vi "getYGAP.vi"(0 "reference":refnum<class "CallNode.lvclass">, 5 "error in (no error)":errorcluster) -> (14 "reference out":refnum<class "CallNode.lvclass">, 15 "CALL_YGAP":i32, 19 "error out":errorcluster)   [LabVIEW 2020, in "CallNode.lvclass"]
doc: "Gets the public YGAP values"
uses:
  <resource>/Framework/Providers/Open_GDS/UML/CallNode_class/CallNode.lvclass
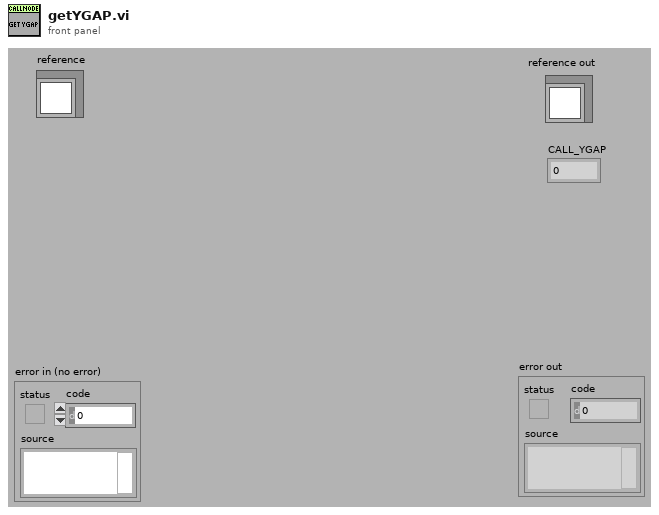
[diagram p1: front panel]
types:
  T1 = typedef "CallNode.lvclass/ClassAttributes.ctl" = cluster{"Base class":T2, "CALL_YGAP":i32}
  T2 = typedef "RectangularNode.lvclass/ClassAttributes.ctl" = cluster{"Base class":T3, "childClassAttribute2":enum16{"Hello", "Goodbye"}}
  T3 = typedef "AbstractNode.lvclass/ClassAttributes.ctl" = cluster{"classAttribute1":bool}
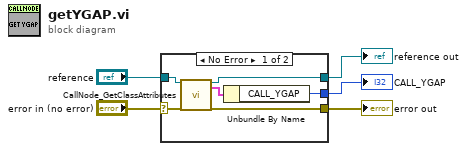
[diagram p0: block diagram]
diagram:
  n1 = case shown="No Error" "error in (no error)" {
    selector: "error in (no error)" -> [w11 w12]
    tunnel: "reference" -> [w10 w13]
    tunnel: [w8 w12] -> w3
    tunnel: [w9 w13] -> w2
    tunnel: [w7 _] -> w1
    frame No Error {
      n2 = call <resource>:"CallNode_GetClassAttributes.vi"("reference in"=w10, "error in (no error)"=w11) -> ("reference out"=w9:refnum<class "CallNode.lvclass">, "Class attribute"=w6:T1, "error out"=w8:errorcluster)  [unwired: 15 out]
      n3 = Unbundle By Name(w6) -> ("CALL_YGAP"=w7:i32)
    }
    frame Error {
    }
  }
  "reference out" <- w2
  "error out" <- w3
  "CALL_YGAP" <- w1
